vi "loglookup.vi"(0 "A/D bits":i32=8, 2 "virtual T/R Pairs":i32=1) -> (3 "Log Lookup":sgl[](array[numeric]), 4 "16 bit scale factor":dbl, 5 "BFormed Bits":dbl, 6 "Minimum dB":dbl format="%#_13g")   [LabVIEW 2022 SP3]
uses:
  Misc Programs/MathOperations/Decimal Rounding.vi
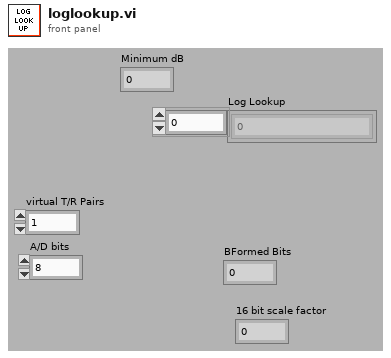
[diagram p1: front panel]
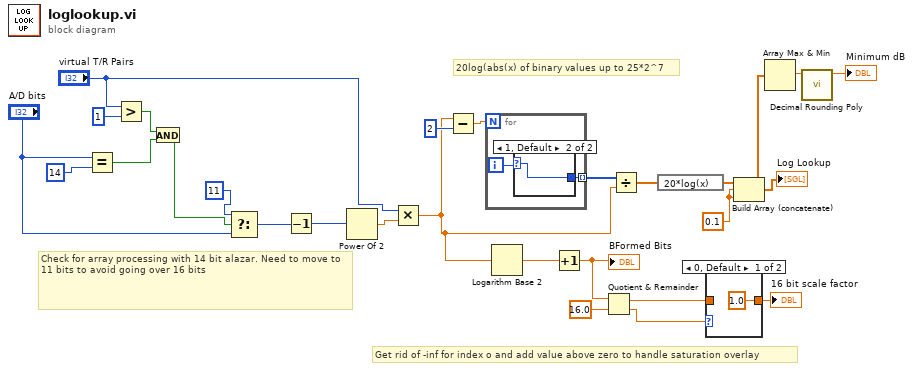
[diagram p0: block diagram]
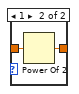
[diagram p2: hidden frame]
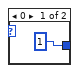
[diagram p3: hidden frame]
diagram:
  w22 = 0.1
  # "Check for array processing with 14 bit alazar. Need to move to 11 bits to avoid going over 16 bits"
  # "Get rid of -inf for index o and add value above zero to handle saturation overlay"
  # "20log(abs(x) of binary values up to 25*2^7"
  n1 = Equal?(x="A/D bits", y=14) -> (x = y?=w8:bool)
  n2 = Greater?(x="virtual T/R Pairs", y=1) -> (0:w9:bool)
  n3 = And(x=w9, y=w8) -> (x .and. y?=w7:bool)
  n4 = Select(t=11, s=w7, f="A/D bits") -> (s? t:f=w4:i32)
  n5 = Decrement(x=w4) -> (x-1=w21:i32)
  n6 = Power Of 2(x=w21) -> (2^x=w20:dbl)
  n7 = Multiply(x="virtual T/R Pairs", y=w20) -> (x*y=w19:dbl)
  n8 = Subtract(x=w19, y=2) -> (x-y=w25:dbl)
  n9 = for {
    N: w25 -> [_]
    tunnel: [w28] -> w27 mode=indexing
    i -> [w29]
    n10 = case shown="1, Default" w29 {
      selector: w29 -> [_ w31]
      tunnel: [1 w31] -> w28
      frame 0 {
      }
      frame 1, Default {
      }
    }
  }
  n11 = Logarithm Base 2(1:w19) -> (0:w18:dbl)
  n12 = Increment(x=w18) -> (x+1=w14:dbl)
  "BFormed Bits" <- w14
  n13 = Quotient & Remainder(x=w14, y=16.0) -> (x-y*floor(x/y)=w16:dbl, floor(x/y)=w13:dbl)
  n14 = Divide(x=w27, y=w19) -> (x/y=w26:dbl[])
  n15 = expression code="20*log(x)"(w26) -> (w23:dbl[])
  n16 = case shown="0, Default" w13 {
    tunnel: w16 -> [_ w34]
    tunnel: [1.0 w33] -> w15
    frame 0, Default {
    }
    frame 1 {
      n17 = Power Of 2(x=w34) -> (2^x=w33:dbl)
    }
  }
  "16 bit scale factor" <- w15
  n18 = Build Array (concatenate)(w23, w22, w22) -> (w3:dbl[])
  "Log Lookup" <- w3
  n19 = Array Max & Min(array=w3) -> (min value=w2:dbl)  [unwired: 3 out]
  n20 = call-poly "Decimal Rounding Poly.vi"("Input"=w2) -> ("Output"=→"Minimum dB":dbl)  [unwired: 10 in]
